vi "Bulk Create.vi"(4 "TypeMap in":refnum<class "TypeMap.lvclass">, 6 "commandTimeout":i32=-1, 8 "error in (no error)":errorcluster, 10 "object in":refnum<class>[](array[class]), 11 "SqlMapper in":refnum<class "SqlMapper.lvclass">) -> (0 "error out":errorcluster, 1 "id":i32[](array[numeric]), 2 "object out":refnum<class>[](array[class]), 3 "SqlMapper out":refnum<class "SqlMapper.lvclass">)   [LabVIEW 2020, in "ORM.lvlib" / "TypeMap.lvclass"]
uses:
  TypeMap.lvclass
  TypeMap.lvclass/TypeMap.ctl
  DbConnection/DbConnection.lvclass
  SqlMapper/SqlMapper.lvclass
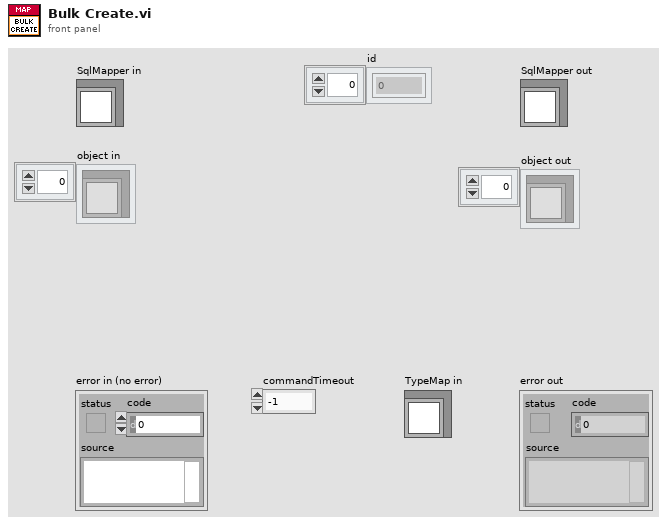
[diagram p1: front panel]
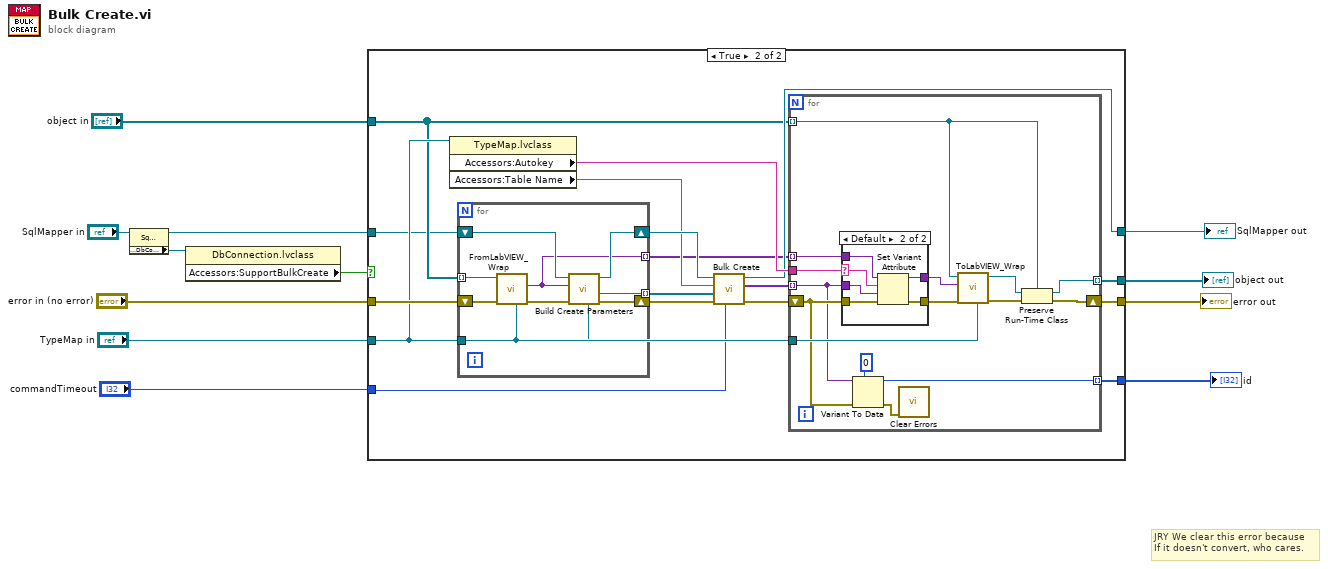
[diagram p0: block diagram]
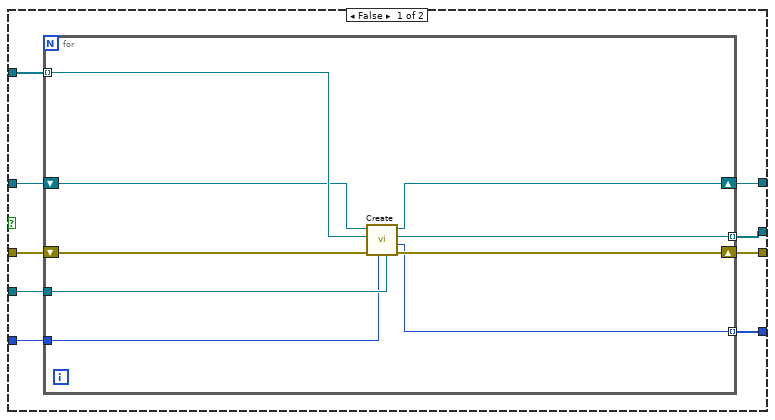
[diagram p2: hidden frame]
diagram:
  # "JRY We clear this error because\nIf it doesn't convert, who cares."
  n1 = property class="SqlMapper.lvclass"(reference="SqlMapper in") -> (reference out=w3:refnum<class "SqlMapper.lvclass">, "Accessors:DbConnection"=w2:refnum<class "DbConnection.lvclass">)  [unwired: 1 in, 1 out]
  n2 = property class="DbConnection.lvclass"(reference=w2) -> ("Accessors:SupportBulkCreate"=w1:bool)  [unwired: 1 in, 2 out]
  n3 = case shown="True" w1 {
    tunnel: "error in (no error)" -> [w21 w45]
    tunnel: "commandTimeout" -> [w14 w31]
    tunnel: [w18 w40] -> w9
    tunnel: [w16 w39] -> w8
    tunnel: [w17 w38] -> w7
    tunnel: "TypeMap in" -> [w15 w36]
    tunnel: "object in" -> [w20 w35]
    tunnel: [w13 w33] -> w4
    tunnel: w3 -> [w19 w32]
    frame False {
      n4 = for {
        tunnel: w20 -> [w29] mode=indexing
        shift-right: [w27] -> w18
        shift-left: w19 -> [w28]
        tunnel: [w26] -> w17 mode=indexing
        shift-right: [w25] -> w16
        shift-left: w21 -> [w30]
        tunnel: w15 -> [w24]
        tunnel: w14 -> [w23]
        tunnel: [w22] -> w13 mode=indexing
        n5 = call-dynamic "Create.vi"("TypeMap in"=w24, "commandTimeout"=w23, "error in (no error)"=w30, "object in"=w29, "SqlMapper in"=w28) -> ("error out"=w25:errorcluster, "id"=w22:i32, "object out"=w26:refnum<class>, "SqlMapper out"=w27:refnum<class "SqlMapper.lvclass">)  [unwired: 3 in]
      }
    }
    frame True {
      n6 = property class="TypeMap.lvclass"(reference=w36) -> ("Accessors:Autokey"=w44:string, "Accessors:Table Name"=w41:string)  [unwired: 1 in, 2 out]
      n7 = for {
        tunnel: [w51] -> w37 mode=indexing
        tunnel: w36 -> [w50]
        tunnel: w35 -> [w49] mode=indexing
        shift-right: [w54] -> w46
        shift-left: w45 -> [w53]
        shift-right: [w55] -> w47
        shift-left: w32 -> [w52]
        tunnel: [w48] -> w34 mode=indexing
        n8 = call "FromLabVIEW_Wrap.vi"("TypeMap in"=w50, "error in (no error)"=w53, "object in"=w49) -> ("error out"=w56:errorcluster, "DbRow"=w51:variant)  [unwired: 7 in]
        n9 = call-dynamic "Build Create Parameters.vi"("TypeMap in"=w50, "error in (no error)"=w56, "object"=w51, "SqlMapper in"=w52) -> ("error out"=w54:errorcluster, "DynamicParameters out"=w48:refnum<class "DynamicParameters.lvclass">, "SqlMapper out"=w55:refnum<class "SqlMapper.lvclass">)  [unwired: 5 in]
      }
      n10 = call "Bulk Create.vi"("commandTimeout"=w31, "error in (no error)"=w46, "DynamicParameters"=w34, "tableName"=w41, "SqlMapper in"=w47) -> ("error out"=w42:errorcluster, "id"=w43:variant[], "SqlMapper out"=w40:refnum<class "SqlMapper.lvclass">)  [unwired: 4 in]
      n11 = for {
        tunnel: w44 -> [w69]
        tunnel: w43 -> [w57] mode=indexing
        tunnel: [w66] -> w38 mode=indexing
        tunnel: w37 -> [w65] mode=indexing
        tunnel: w36 -> [w64]
        tunnel: w35 -> [w63] mode=indexing
        shift-right: [w68] -> w39
        shift-left: w42 -> [w60]
        tunnel: [w58] -> w33 mode=indexing
        n12 = case shown="Default" w69 {
          selector: w69 -> [_ w77]
          tunnel: [w73 w79] -> w70
          tunnel: w65 -> [w72 w78]
          tunnel: w60 -> [w73 w74]
          tunnel: w57 -> [_ w75]
          tunnel: [w72 w76] -> w62
          frame "" {
          }
          frame Default {
            n13 = Set Variant Attribute(Variant=w78, name=w77, value=w75, error in=w74) -> (Variant out=w76:variant, error out=w79:errorcluster)  [unwired: 1 out]
          }
        }
        n14 = Variant To Data(error in=w60, type=0, Variant=w57) -> (data=w58:i32, error out=w61:errorcluster)
        n15 = call <vilib>:"Clear Errors.vi"("error in (no error)"=w61) -> ()  [unwired: 5 in, 2 out]
        n16 = call "ToLabVIEW_Wrap.vi"("TypeMap in"=w64, "error in (no error)"=w70, "DbRow"=w62, "TargetObject In"=w63) -> ("error out"=w71:errorcluster, "Object Out"=w67:refnum<class>)  [unwired: 6 in]
        n17 = Preserve Run-Time Class(object in=w67, error in=w71, 2:w63) -> (object out=w66:refnum<class>, error out=w68:errorcluster)
      }
    }
  }
  "error out" <- w8
  "SqlMapper out" <- w9
  "object out" <- w7
  "id" <- w4
